vi "about_window.vi"(8 "error_in":errorcluster caption="(ий)error_in", 10 "lines_to_bold":i32[](array[numeric])=[0, 3] caption="(ий)lines_to_bold", 11 "about_string":string caption="(ий)about_string") -> (0 "error_out":errorcluster caption="(ий)error_out")   [LabVIEW 2020]
doc: "This VI displays informations about program, contained in about_string, bolding some of the lines in message. If you want to customize look of about message, you can do it here."
uses:
  AULocalize/SubVIs/RegisterVI.vi
panel:
  out "About":string=" Programie"
  in  "OK":bool caption="(ий)OK"
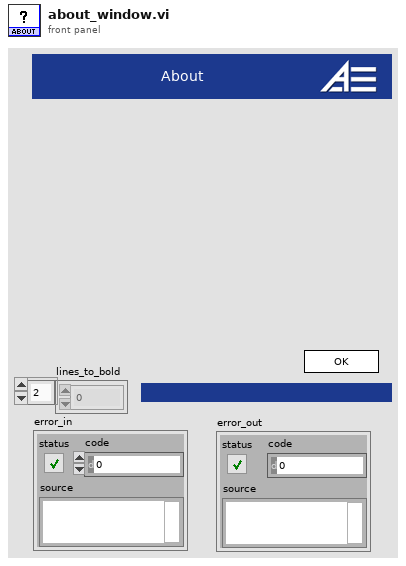
[diagram p1: front panel]
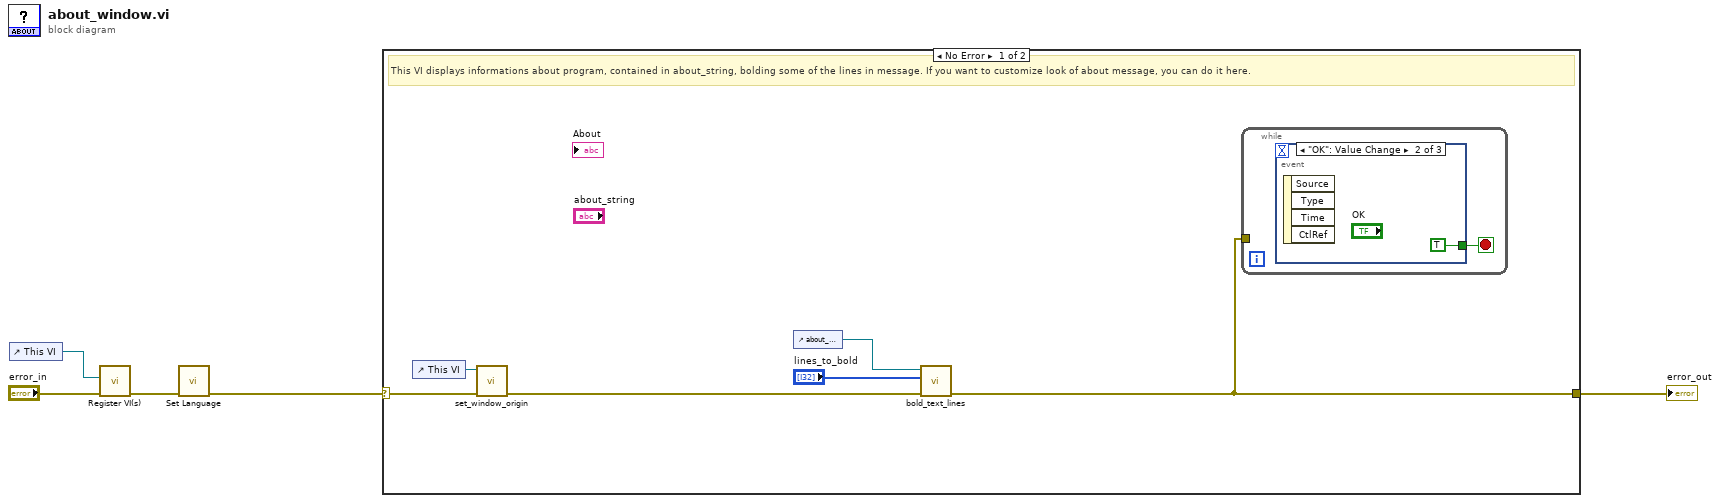
[diagram p0: block diagram]
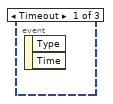
[diagram p2: hidden frame]
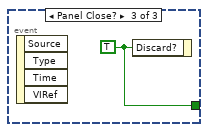
[diagram p3: hidden frame]
diagram:
  n1 = control-ref of="This VI"() -> (w1:refnum<vi>)
  n2 = call-poly "Register VI(s).vi"("error in"="error_in", "VI Ref"=w1) -> ("error out"=w3:errorcluster)  [unwired: 8 in, 1 out]
  n3 = call "Set Language.vi"("error in"=w3) -> ("error out"=w2:errorcluster)  [unwired: 9 in, 1 out]
  n4 = case shown="No Error" w2 {
    selector: w2 -> [w6 w15]
    tunnel: [w7 w15] -> w5
    frame No Error {
      # "This VI displays informations about program, contained in about_string, bolding some of the lines in message. If you want to customize look of about message, you can do it here."
      n5 = control-ref of="This VI"() -> (w10:refnum<vi>)
      n6 = call "set_window_origin.vi"("error_in"=w6, "this_vi_reference"=w10) -> ("error_out"=w9:errorcluster)  [unwired: 9 in]
      n7 = control-ref of="about_string"() -> (w8:refnum<vi>)
      n8 = call "bold_text_lines.vi"("error in (no error)"=w9, "Lines to bold"="lines_to_bold", "String to bold reference"=w8) -> ("error out"=w7:errorcluster)  [unwired: 8 in]
      n9 = while {
        tunnel: w7 -> [_]
        stop <- w12 stop-if-true
        n10 = event shown="[1] \"OK\": Value Change" {
          selector: _ -> [_ _ _]
          dyn-events: _ -> [_ _ _]
          timeout: _ -> [_ _ _]
          tunnel: [_ TRUE ("stop") w14] -> w12
          event Timeout {
            n11 = event-data() -> ()  [unwired: 1 in, 2 out]
          }
          event "OK": Value Change {
            n12 = event-data() -> ()  [unwired: 1 in, 4 out]
          }
          event Panel Close? {
            w14 = TRUE ("Discard?")
            n13 = event-data() -> ()  [unwired: 1 in, 4 out]
            n14 = event-data("Discard?"=w14) -> ()  [unwired: 1 in, 1 out]
          }
        }
      }
    }
    frame Error {
      # "This VI displays informations about program, contained in about_string, bolding some of the lines in message. If you want to customize look of about message, you can do it here."
    }
  }
  "error_out" <- w5
